vi "Q3.vi"() -> ()   [LabVIEW 2018]
uses:
  <vilib>/Analysis/NI_AALBase.lvlib
panel:
  in  "stop 2":bool
  in  "amplitude of the waveform  2":dbl(knob) scale=0.0..180.0
  in  "Frequency of the waveform 2":dbl(knob) scale=0.0..180.0
  out "Sine":dynamicdata(graph)
  in  "stop":bool
  in  "amplitude of the waveform":dbl(knob) scale=0.0..180.0
  in  "Frequency of the waveform":dbl(knob) scale=0.0..180.0
  out "Waveform Chart":dbl[](graph)
  # "Question 3"
  # "First way"
  # "second way"
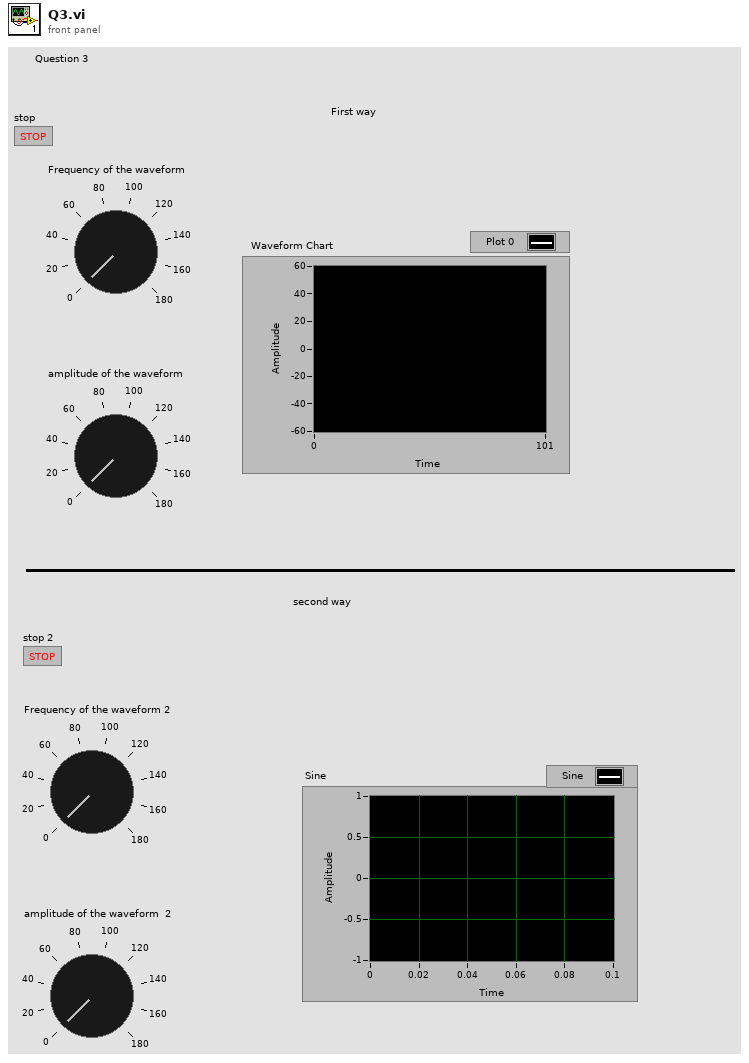
[diagram p1: front panel]
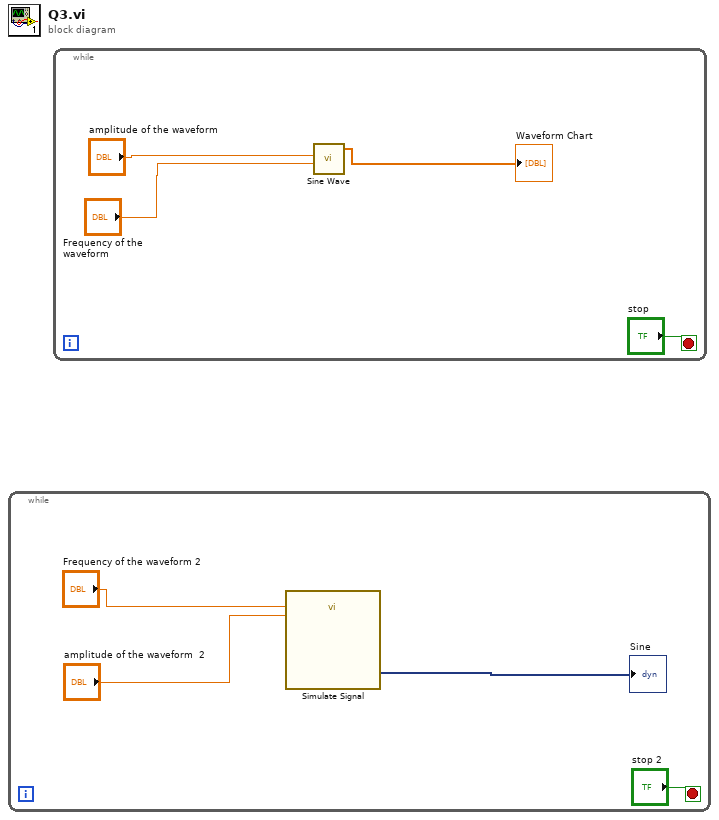
[diagram p0: block diagram]
diagram:
  n1 = while {
    stop <- "stop 2" stop-if-true
    n2 = call "Simulate Signal"("Frequency"="Frequency of the waveform 2", "Amplitude"="amplitude of the waveform  2") -> ("Sine"=→"Sine":dynamicdata)  [unwired: 12 in, 1 out]
  }
  n3 = while {
    stop <- "stop" stop-if-true
    n4 = call <vilib>:"Sine Wave.vi"("amplitude"="amplitude of the waveform", "frequency"="Frequency of the waveform") -> ("sine wave"=→"Waveform Chart":dbl[])  [unwired: 3 in, 2 out]
  }
